vi "ConfigureClk.vi"(8 "error in (no error)":errorcluster, 10 "ClkName":string, 11 "PXI_MultiTrig in":refnum<class "PXI_MultiTrig.lvclass">) -> (0 "error out":errorcluster, 3 "PXI_MultiTrig out":refnum<class "PXI_MultiTrig.lvclass">)   [LabVIEW 2018, in "SyncPlugins.lvlib" / "PXI_MultiTrig.lvclass"]
uses:
  PXI_MultiTrig.lvclass
  X:/Projects/PMUCal/Modules/Sync/SyncPlugins/SyncPluginBase/SyncPluginBase.lvclass
  Typedefs/clClocks.ctl
  PXI_MultiTrig.lvclass/PXI_MultiTrig.ctl
  Accessors/Read TimingSession.vi
  Accessors/Read RefClkSession.vi
  SyncPluginBase/Accessors/Read Clocks.vi
  <vilib>/Utility/error.llb/Error Cluster From Error Code.vi
  SyncPluginBase/Accessors/Write Clocks.vi
  <instrlib>/niSync/niSync.llb/niSync Create Clock (Frequency).vi
  <vilib>/ErrorRing/Error Ring.xnode
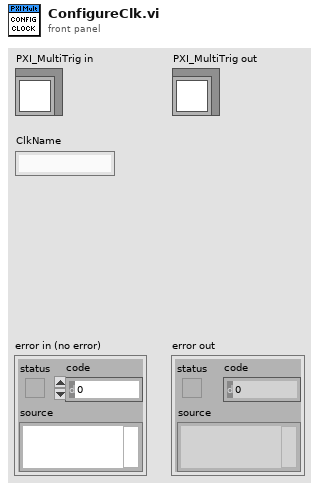
[diagram p1: front panel]
types:
  T1 = typedef "SyncPlugins.lvlib/PXI_MultiTrig.lvclass/clClocks.ctl" = cluster{"Name":string, "RefClk":string, "ClkTerminal":string, "Frequency":dbl, "DutyCycle":dbl, "ClkType":string, "Initiated":bool, "TrigTime":bool, "Delay":dbl}
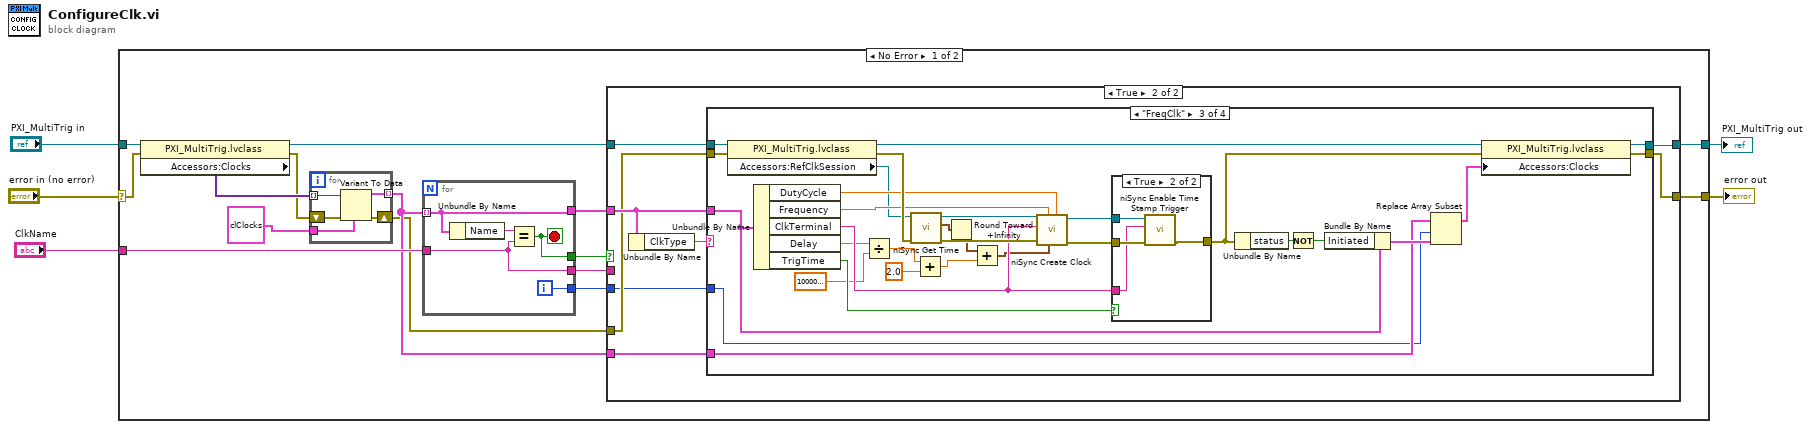
[diagram p0: block diagram]
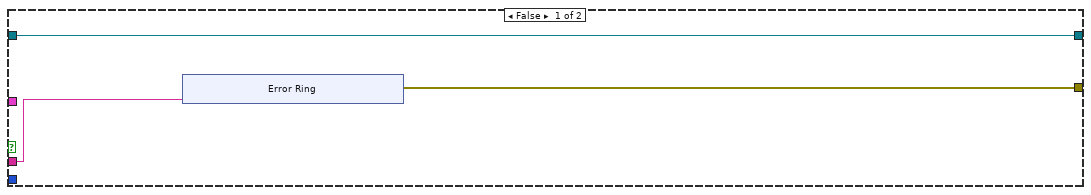
[diagram p2: hidden frame]
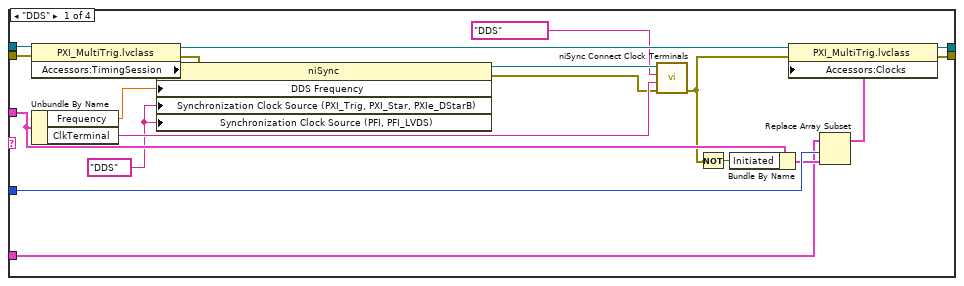
[diagram p3: hidden frame]
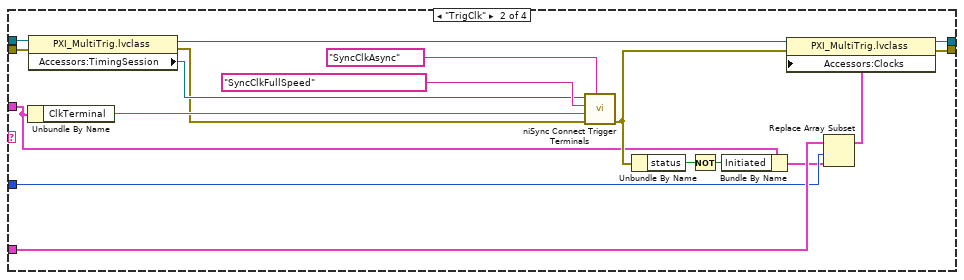
[diagram p4: hidden frame]
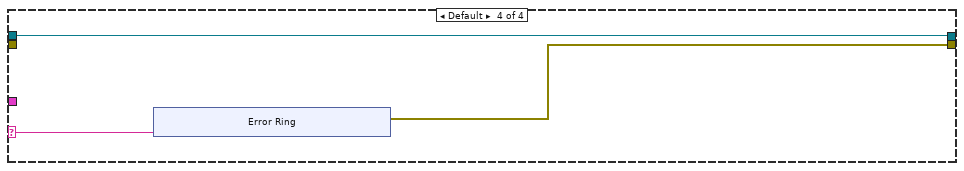
[diagram p6: hidden frame]
diagram:
  n1 = case shown="No Error" "error in (no error)" {
    selector: "error in (no error)" -> [w19 w134]
    tunnel: [w12 w134] -> w4
    tunnel: [w13 w133] -> w2
    tunnel: "PXI_MultiTrig in" -> [w20 w133]
    tunnel: "ClkName" -> [w18 _]
    frame No Error {
      n2 = property class="PXI_MultiTrig.lvclass"(reference=w20, error in=w19) -> (reference out=w14:refnum<class "PXI_MultiTrig.lvclass">, error out=w7:errorcluster, "Accessors:Clocks"=w10:variant[])
      n3 = for {
        tunnel: w10 -> [w25] mode=indexing
        tunnel: [w24] -> w9 mode=indexing
        shift-right: [w22] -> w8
        shift-left: w7 -> [w23]
        tunnel: T1 {"Name"="", "RefClk"="/PXI1Slot7/PFI1", "ClkTerminal"="PXI_Star4", "Frequency"=0.0, "DutyCycle"=0.0, "ClkType"="", "Initiated"=FALSE, "TrigTime"=FALSE, "Delay"=0.0} ("clClocks") -> [w21]
        n4 = Variant To Data(error in=w23, type=w21, Variant=w25) -> (data=w24:T1, error out=w22:errorcluster)
      }
      n5 = for {
        tunnel: w9 -> [w131] mode=indexing
        tunnel: w18 -> [w129]
        tunnel: [w131] -> w15
        tunnel: [w130] -> w17
        tunnel: [w129] -> w16
        tunnel: [w128] -> w11
        i -> [w128]
        stop <- w130 stop-if-true
        n6 = Unbundle By Name(w131) -> ("Name"=w132:string)
        n7 = Equal?(x=w132, y=w129) -> (x = y?=w130:bool)
      }
      n8 = case shown="True" w17 {
        tunnel: w8 -> [_ w40]
        tunnel: w16 -> [w28 _]
        tunnel: w15 -> [_ w42]
        tunnel: w14 -> [w27 w41]
        tunnel: [w27 w39] -> w13
        tunnel: [w26 w38] -> w12
        tunnel: w11 -> [_ w37]
        tunnel: w9 -> [_ w36]
        frame False {
          n9 = xnode "Error Ring"("parameter 0"=w28) -> ("error out"=w26:errorcluster)
        }
        frame True {
          n10 = Unbundle By Name(w42) -> ("ClkType"=w43:string)
          n11 = case shown="\"FreqClk\"" w43 {
            selector: w43 -> [_ _ _ w120]
            tunnel: w42 -> [w54 w65 w96 _]
            tunnel: w40 -> [w61 w77 w111 _]
            tunnel: [w56 w73 w110 w119] -> w38
            tunnel: w41 -> [w62 w78 w112 w118]
            tunnel: [w57 w74 w109 w118] -> w39
            tunnel: w37 -> [w53 w67 w97 _]
            tunnel: w36 -> [w51 w68 w104 _]
            frame "DDS" {
              w44 = "DDS" ("Synchronization Clock Properties:Synchronization Clock Source (PXI_Trig, PXI_Star, PXIe_DStarB)")
              n12 = property class="PXI_MultiTrig.lvclass"(reference=w62, error in=w61) -> (reference out=w58:refnum<class "PXI_MultiTrig.lvclass">, error out=w59:errorcluster, "Accessors:TimingSession"=w60:refnum<k15>)
              n13 = Unbundle By Name(w54) -> ("Frequency"=w63:dbl, "ClkTerminal"=w47:string)
              n14 = property class="niSync"(reference=w60, error in=w59, "DDS Frequency"=w63, "Synchronization Clock Source (PXI_Trig, PXI_Star, PXIe_DStarB)"=w44, "Synchronization Clock Source (PFI, PFI_LVDS)"=w44) -> (reference out=w49:refnum<k15>, error out=w46:errorcluster)
              n15 = call <instrlib>:"niSync Connect Clock Terminals.vi"("error in (no error)"=w46, "destination terminal"=w47, "source terminal"="DDS", "instrument handle"=w49) -> ("error out"=w45:errorcluster)  [unwired: 6 in, 1 out]
              n16 = Not(x=w45) -> (.not. x?=w55:bool)
              n17 = Bundle By Name(cluster=w54, "Initiated"=w55) -> (w52:T1)
              n18 = Replace Array Subset(array=w51, new element=w52, index=w53) -> (w50:T1[])
              n19 = property class="PXI_MultiTrig.lvclass"(reference=w58, error in=w45, "Accessors:Clocks"=w50) -> (reference out=w57:refnum<class "PXI_MultiTrig.lvclass">, error out=w56:errorcluster)
            }
            frame "TrigClk" {
              n20 = Unbundle By Name(w65) -> ("ClkTerminal"=w81:string)
              n21 = property class="PXI_MultiTrig.lvclass"(reference=w78, error in=w77) -> (reference out=w72:refnum<class "PXI_MultiTrig.lvclass">, error out=w75:errorcluster, "Accessors:TimingSession"=w76:refnum<k15>)
              n22 = call <instrlib>:"niSync Connect Trigger Terminals.vi"("synchronization clock"="SyncClkAsync", "error in (no error)"=w75, "destination terminal"=w81, "source terminal"="SyncClkFullSpeed", "instrument handle"=w76) -> ("error out"=w69:errorcluster)  [unwired: 5 in, 1 out]
              n23 = Unbundle By Name(w69) -> ("status"=w70:bool)
              n24 = Not(x=w70) -> (.not. x?=w71:bool)
              n25 = Bundle By Name(cluster=w65, "Initiated"=w71) -> (w66:T1)
              n26 = Replace Array Subset(array=w68, new element=w66, index=w67) -> (w64:T1[])
              n27 = property class="PXI_MultiTrig.lvclass"(reference=w72, error in=w69, "Accessors:Clocks"=w64) -> (reference out=w74:refnum<class "PXI_MultiTrig.lvclass">, error out=w73:errorcluster)
            }
            frame "FreqClk" {
              n28 = property class="PXI_MultiTrig.lvclass"(reference=w112, error in=w111) -> (reference out=w108:refnum<class "PXI_MultiTrig.lvclass">, error out=w101:errorcluster, "Accessors:RefClkSession"=w82:refnum<k15>)
              n29 = Unbundle By Name(w96) -> ("DutyCycle"=w99:dbl, "Frequency"=w98:dbl, "ClkTerminal"=w95:string, "Delay"=w89:dbl, "TrigTime"=w91:bool)
              n30 = Divide(x=w89, y=1000000.0) -> (x/y=w87:dbl)
              n31 = call <instrlib>:"niSync Get Time.vi"("error in (no error)"=w101, "instrument handle"=w82) -> ("error out"=w100:errorcluster, "time"=w85:timestamp, "instrument handle out"=w102:refnum<k15>)  [unwired: 5 in]
              n32 = Add(x=w87, y=2.0) -> (x+y=w90:dbl)
              n33 = Round Toward +Infinity(x=w85) -> (ceil(x): smallest int >= x=w84:timestamp)
              n34 = Add(x=w84, y=w90) -> (x+y=w83:timestamp)
              n35 = call-poly <instrlib>:"niSync Create Clock.vi"("duty cycle"=w99, "start time"=w83, "frequency"=w98, "error in (no error)"=w100, "terminal"=w95, "instrument handle"=w102) -> ("error out"=w94:errorcluster, "instrument handle out"=w92:refnum<k15>)  [unwired: 2 in, 2 out]
              n36 = case shown="True" w91 {
                tunnel: w95 -> [_ w115]
                tunnel: w94 -> [w113 w117]
                tunnel: [w113 w116] -> w93
                tunnel: w92 -> [_ w114]
                frame False {
                }
                frame True {
                  n37 = call <instrlib>:"niSync Enable Time Stamp Trigger.vi"("error in (no error)"=w117, "terminal"=w115, "instrument handle"=w114) -> ("error out"=w116:errorcluster)  [unwired: 6 in, 1 out]
                }
              }
              n38 = Unbundle By Name(w93) -> ("status"=w106:bool)
              n39 = Not(x=w106) -> (.not. x?=w105:bool)
              n40 = Bundle By Name(cluster=w96, "Initiated"=w105) -> (w107:T1)
              n41 = Replace Array Subset(array=w104, new element=w107, index=w97) -> (w103:T1[])
              n42 = property class="PXI_MultiTrig.lvclass"(reference=w108, error in=w93, "Accessors:Clocks"=w103) -> (reference out=w109:refnum<class "PXI_MultiTrig.lvclass">, error out=w110:errorcluster)
            }
            frame Default {
              n43 = xnode "Error Ring"("parameter 0"=w120) -> ("error out"=w119:errorcluster)
            }
          }
        }
      }
    }
    frame Error {
    }
  }
  "error out" <- w4
  "PXI_MultiTrig out" <- w2
